vi "Main.vi"() -> ()   [LabVIEW 2013]
doc: "This template is for the Queued Message Handler design pattern.\n\nThe Event Handling Loop generates messages based on user interface actions.\n\nThe Message Handling Loop processes messages generated by the Event Handling Loop, or by other messages. The messages are string values, so new messages can be added easily to the Message Cases case structure in the Message Handling Loop. Each message cluster can also provide an optional value for Message Data, which is a variant that can be converted to whatever message-specific data is required."
uses:
  controls/UI Data.ctl
  support/Message Queue/Enqueue Message (Single).vi
  support/Message Queue/Enqueue Message (Array).vi
  <vilib>/Utility/error.llb/Error Cluster From Error Code.vi
  <vilib>/ErrorRing/Error Ring.xnode
  support/Message Queue/Message Queue.lvlib
  support/User Event - Stop/User Event - Stop.lvlib
panel:
  out "Display <Replace Me>":string
  in  "Do Something Else <Replace Me>":bool
  in  "Do Something <Replace Me>":bool
  in  "Exit":bool
  # "These controls have associated \"Value Changed\" events configured in the Event Structure on the diagram.\n\nReplace them (and reconfigure the Event Structure) with the controls you need for your application."
  # "This template is for the Queued Message Handler design pattern.\n\nSee the block diagram for more information on how to use this template."
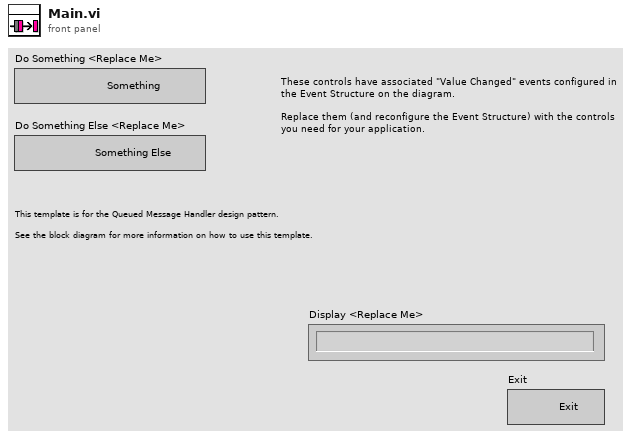
[diagram p1: front panel]
types:
  T1 = typedef "UI Data.ctl" = cluster{"Boolean <Replace Me>":bool, "String <Replace Me>":string, "Numeric <Replace Me>":dbl, "Do Something Ref":refnum<vi>, "Do Something Else Ref":refnum<vi>, "Data Display Ref":refnum<vi>, "Exit Button Ref":refnum<vi>}
  T2 = typedef "Message Queue.lvlib/All Message Queues.ctl" = cluster{"UI":refnum<queue>}
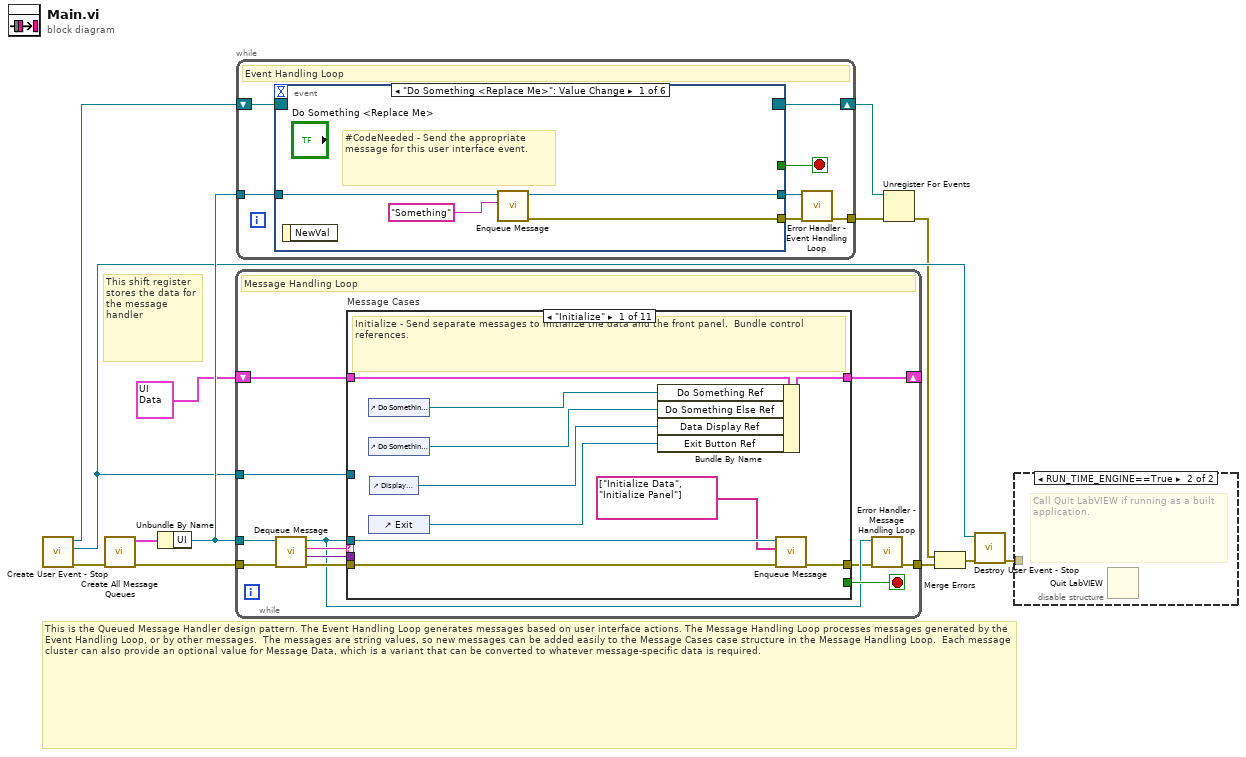
[diagram p0: block diagram]
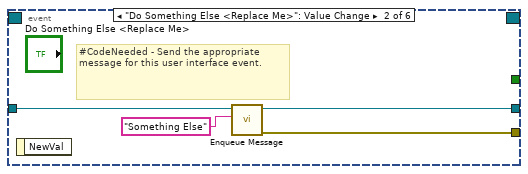
[diagram p3: hidden frame]
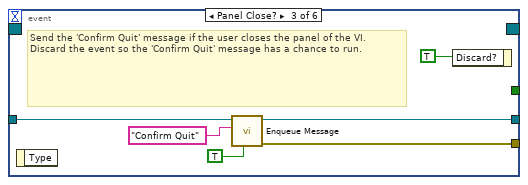
[diagram p4: hidden frame]
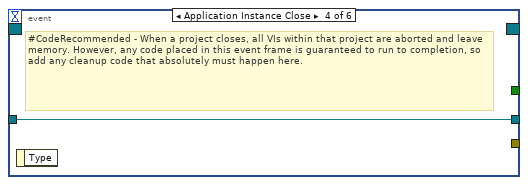
[diagram p5: hidden frame]
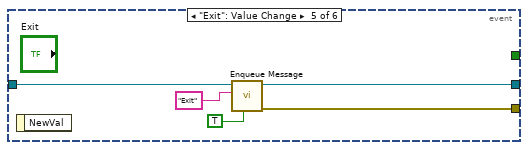
[diagram p6: hidden frame]
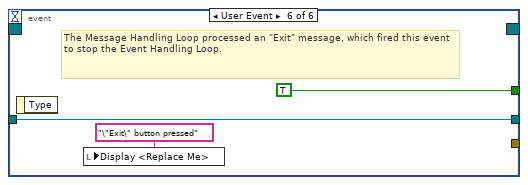
[diagram p7: hidden frame]
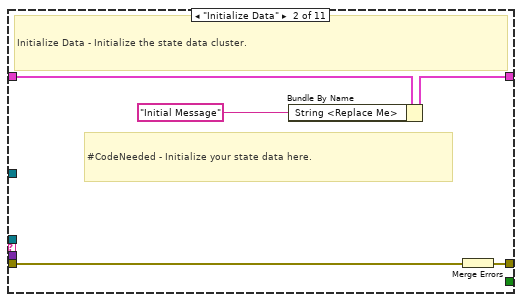
[diagram p8: hidden frame]
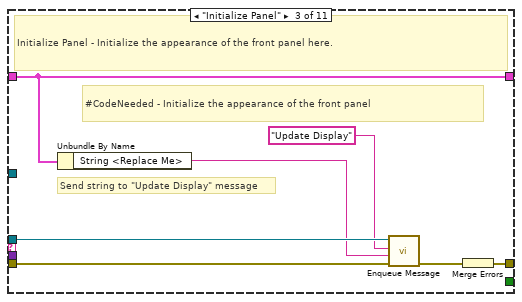
[diagram p9: hidden frame]
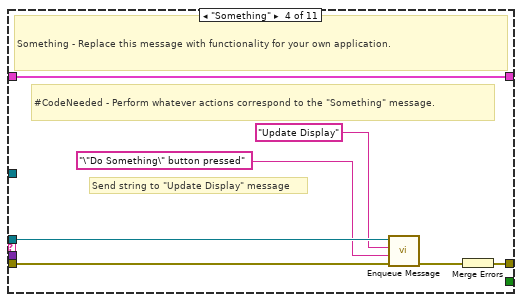
[diagram p10: hidden frame]
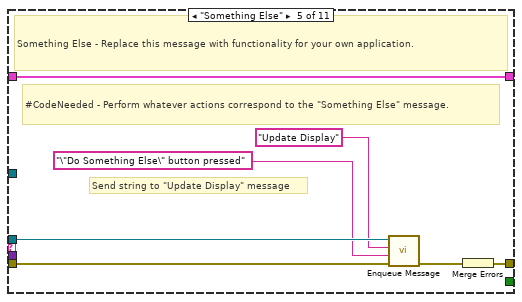
[diagram p11: hidden frame]
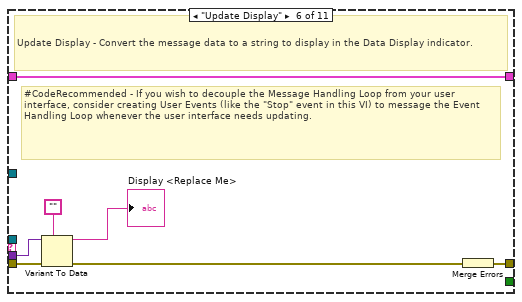
[diagram p12: hidden frame]
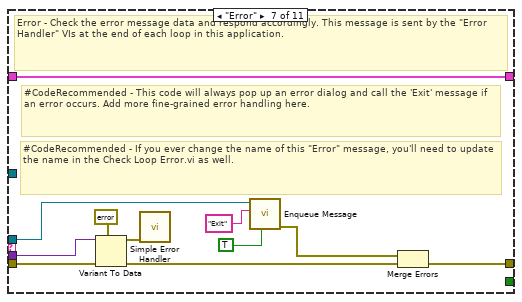
[diagram p13: hidden frame]
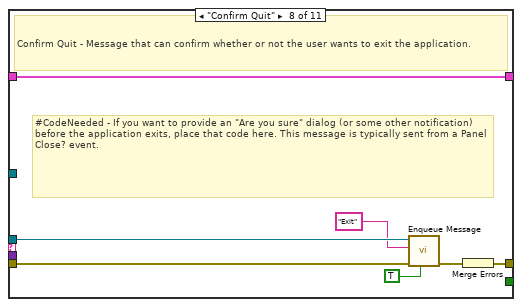
[diagram p14: hidden frame]
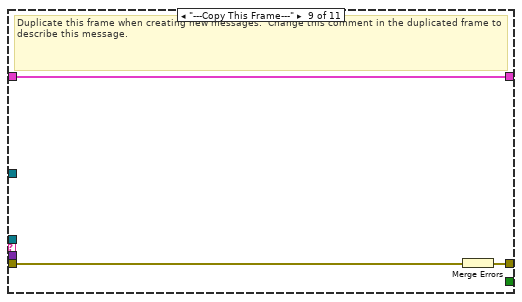
[diagram p15: hidden frame]
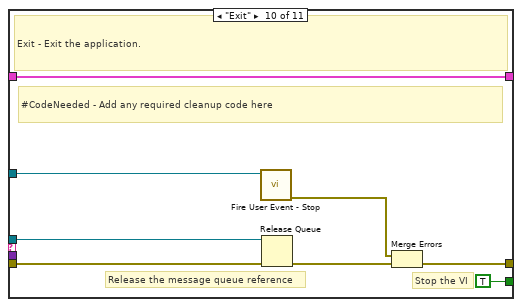
[diagram p16: hidden frame]
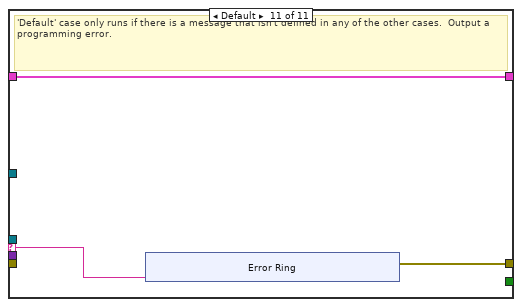
[diagram p17: hidden frame]
diagram:
  # "This is the Queued Message Handler design pattern. The Event Handling Loop generates messages based on user interface actions. The Message Handling Loop processes messages generated by the Event Handling Loop, or by other messages.  The messages are string values, so new messages can be added easily to the Message Cases case structure in the Message Handling Loop.  Each message cluster can also provide an optional value for Message Data, which is a variant that can be converted to whatever message-specific data is required."
  # "This shift register stores the data for the message handler"
  n1 = call "Create User Event - Stop.vi"() -> ("error out"=w8:errorcluster, "User Event - Stop"=w6:refnum<user-event>, "Stop Event Registration Refnum"=w9:refnum<event-registration>)  [unwired: 9 in]
  n2 = call "Create All Message Queues.vi"("error in (no error)"=w8) -> ("error out"=w13:errorcluster, "Message Queues out"=w12:T2)  [unwired: 9 in]
  n3 = Unbundle By Name(w12) -> ("UI"=w10:refnum<queue>)
  n4 = while {
    tunnel: w10 -> [w17]
    shift-right: [w24] -> _
    shift-left: T1 {"Boolean <Replace Me>"=FALSE, "String <Replace Me>"="", "Numeric <Replace Me>"=0.0, "Do Something Ref"=refnum, "Do Something Else Ref"=refnum, "Data Display Ref"=refnum, "Exit Button Ref"=refnum} ("Data Cluster") -> [w25]
    tunnel: w6 -> [w22]
    tunnel: w13 -> [w21]
    tunnel: [w15] -> w11
    stop <- w23 stop-if-true
    # "Message Handling Loop"
    n5 = call "Dequeue Message.vi"("error in (no error)"=w21, "Message Queue"=w17) -> ("error out"=w20:errorcluster, "Message Data"=w18:variant, "Message"=w19:string, "dup Message Queue"=w16:refnum<queue>)  [unwired: 6 in]
    n6 = case "Message Cases" shown="\"Initialize\"" w19 {
      selector: w19 -> [_ _ _ _ _ _ _ _ _ _ w98]
      tunnel: w16 -> [w33 _ w44 w50 w57 _ w71 w82 _ w97 _]
      tunnel: w20 -> [w34 w40 w45 w52 w59 w66 w79 w86 w89 w92 _]
      tunnel: [w35 w36 w46 w53 w60 w67 w72 w84 w87 w93 w99] -> w14
      tunnel: w25 -> [w32 w39 w47 w54 w61 w68 w78 w85 w88 w96 w100]
      tunnel: [w31 w38 w47 w54 w61 w68 w78 w85 w88 w96 w100] -> w24
      tunnel: [_ _ _ _ _ _ _ _ _ TRUE _] -> w23
      tunnel: w18 -> [_ _ _ _ _ w65 w77 _ _ _ _]
      tunnel: w22 -> [_ _ _ _ _ _ _ _ _ w91 _]
      frame "Initialize" {
        # "Initialize - Send separate messages to initialize the data and the front panel.  Bundle control references."
        n7 = control-ref of="Do Something <Replace Me>"() -> (w30:refnum<vi>)
        n8 = control-ref of="Do Something Else <Replace Me>"() -> (w29:refnum<vi>)
        n9 = control-ref of="Exit"() -> (w27:refnum<vi>)
        n10 = control-ref of="Display <Replace Me>"() -> (w28:refnum<vi>)
        n11 = Bundle By Name(cluster=w32, "Do Something Ref"=w30, "Do Something Else Ref"=w29, "Data Display Ref"=w28, "Exit Button Ref"=w27) -> (w31:T1)
        n12 = call-poly "Enqueue Message.vi"("error in (no error)"=w34, "Message Array"=string[] ["Initialize Data", "Initialize Panel"], "Message Queue"=w33) -> ("error out"=w35:errorcluster)  [unwired: 7 in, 1 out]
      }
      frame "Initialize Data" {
        # "#CodeNeeded - Initialize your state data here."
        # "Initialize Data - Initialize the state data cluster."
        n13 = Bundle By Name(cluster=w39, "String <Replace Me>"="Initial Message" ("Initial Message")) -> (w38:T1)
        n14 = Merge Errors(w40) -> (w36:errorcluster)
      }
      frame "Initialize Panel" {
        # "Send string to \"Update Display\" message"
        # "#CodeNeeded - Initialize the appearance of the front panel"
        # "Initialize Panel - Initialize the appearance of the front panel here."
        n15 = Unbundle By Name(w47) -> ("String <Replace Me>"=w41:string)
        n16 = call-poly "Enqueue Message.vi"("error in (no error)"=w45, "Message Data"=w41, "Message"="Update Display", "Message Queue"=w44) -> ("error out"=w43:errorcluster)  [unwired: 6 in, 1 out]
        n17 = Merge Errors(w43) -> (w46:errorcluster)
      }
      frame "Something" {
        # "Send string to \"Update Display\" message"
        # "#CodeNeeded - Perform whatever actions correspond to the \"Something\" message."
        # "Something - Replace this message with functionality for your own application."
        n18 = call-poly "Enqueue Message.vi"("error in (no error)"=w52, "Message Data"="\"Do Something\" button pressed" ("\"Do Something\" button pressed"), "Message"="Update Display", "Message Queue"=w50) -> ("error out"=w51:errorcluster)  [unwired: 6 in, 1 out]
        n19 = Merge Errors(w51) -> (w53:errorcluster)
      }
      frame "Something Else" {
        # "Send string to \"Update Display\" message"
        # "#CodeNeeded - Perform whatever actions correspond to the \"Something Else\" message."
        # "Something Else - Replace this message with functionality for your own application."
        n20 = call-poly "Enqueue Message.vi"("error in (no error)"=w59, "Message Data"="\"Do Something Else\" button pressed" ("\"Do Something Else\" button pressed"), "Message"="Update Display", "Message Queue"=w57) -> ("error out"=w58:errorcluster)  [unwired: 6 in, 1 out]
        n21 = Merge Errors(w58) -> (w60:errorcluster)
      }
      frame "Update Display" {
        # "#CodeRecommended - If you wish to decouple the Message Handling Loop from your user interface, consider creating User Events (like the \"Stop\" event in this VI) to message the Event Handling Loop whenever the user interface needs updating."
        # "Update Display - Convert the message data to a string to display in the Data Display indicator."
        n22 = Variant To Data(error in=w66, type="", Variant=w65) -> (data=→"Display <Replace Me>":string, error out=w63:errorcluster)
        n23 = Merge Errors(w63) -> (w67:errorcluster)
      }
      frame "Error" {
        # "#CodeRecommended - If you ever change the name of this \"Error\" message, you'll need to update the name in the Check Loop Error.vi as well."
        # "#CodeRecommended - This code will always pop up an error dialog and call the 'Exit' message if an error occurs. Add more fine-grained error handling here."
        # "Error - Check the error message data and respond accordingly. This message is sent by the \"Error Handler\" VIs at the end of each loop in this application."
        n24 = Variant To Data(error in=w79, type=errorcluster {"status"=FALSE, "code"=0, "source"=""} ("error constant"), Variant=w77) -> (data=w75:errorcluster, error out=w74:errorcluster)
        n25 = call <vilib>:"Simple Error Handler.vi"("error in (no error)"=w75) -> ()  [unwired: 4 in, 5 out]
        n26 = call-poly "Enqueue Message.vi"("Priority Message? (F)"=TRUE, "Message"="Exit", "Message Queue"=w71) -> ("error out"=w73:errorcluster)  [unwired: 7 in, 1 out]
        n27 = Merge Errors(w73, w74) -> (w72:errorcluster)
      }
      frame "Confirm Quit" {
        # "#CodeNeeded - If you want to provide an \"Are you sure\" dialog (or some other notification) before the application exits, place that code here. This message is typically sent from a Panel Close? event."
        # "Confirm Quit - Message that can confirm whether or not the user wants to exit the application."
        n28 = call-poly "Enqueue Message.vi"("Priority Message? (F)"=TRUE, "error in (no error)"=w86, "Message"="Exit", "Message Queue"=w82) -> ("error out"=w83:errorcluster)  [unwired: 6 in, 1 out]
        n29 = Merge Errors(w83) -> (w84:errorcluster)
      }
      frame "---Copy This Frame---" {
        # "Duplicate this frame when creating new messages.  Change this comment in the duplicated frame to describe this message."
        n30 = Merge Errors(w89) -> (w87:errorcluster)
      }
      frame "Exit" {
        # "Stop the VI"
        # "Release the message queue reference"
        # "#CodeNeeded - Add any required cleanup code here"
        # "Exit - Exit the application."
        n31 = call "Fire User Event - Stop.vi"("User Event - Stop"=w91) -> ("error out"=w90:errorcluster)  [unwired: 10 in]
        n32 = Release Queue(queue=w97, error in (no error)=w92) -> (error out=w94:errorcluster)  [unwired: 1 in, 2 out]
        n33 = Merge Errors(w90, w94) -> (w93:errorcluster)
      }
      frame Default {
        # "'Default' case only runs if there is a message that isn't defined in any of the other cases.  Output a programming error."
        n34 = xnode "Error Ring"("parameter 0"=w98) -> ("error out"=w99:errorcluster)
      }
    }
    n35 = call "Error Handler - Message Handling Loop.vi"("error in (no error)"=w14, "Message Queue"=w16) -> ("dup error in"=w15:errorcluster)  [unwired: 8 in, 1 out]
  }
  n36 = while {
    tunnel: w10 -> [w114]
    shift-right: [w112] -> w4
    shift-left: w9 -> [w113]
    tunnel: [w108] -> w1
    stop <- w110 stop-if-true
    # "Event Handling Loop"
    n37 = event shown="[0] \"Do Something <Replace Me>\": Value Change" {
      selector: w113 -> [_ _ _ _ _ _]
      dyn-events: [_ _ _ _ _ _] -> w112
      timeout: _ -> [_ _ _ _ _ _]
      tunnel: [_ _ _ _ _ TRUE ("Discard?")] -> w110
      tunnel: w114 -> [w118 w122 w127 w129 w134 w137]
      tunnel: [w115 w119 w126 _ w133 _] -> w111
      tunnel: [w117 w121 w125 w129 w132 w137] -> w109
      event "Do Something <Replace Me>": Value Change {
        # "#CodeNeeded - Send the appropriate message for this user interface event."
        n38 = event-data() -> ()  [unwired: 1 in, 1 out]
        n39 = call-poly "Enqueue Message.vi"("Message"="Something", "Message Queue"=w118) -> ("error out"=w115:errorcluster, "dup Message Queue"=w117:refnum<queue>)  [unwired: 8 in]
      }
      event "Do Something Else <Replace Me>": Value Change {
        # "#CodeNeeded - Send the appropriate message for this user interface event."
        n40 = event-data() -> ()  [unwired: 1 in, 1 out]
        n41 = call-poly "Enqueue Message.vi"("Message"="Something Else", "Message Queue"=w122) -> ("error out"=w119:errorcluster, "dup Message Queue"=w121:refnum<queue>)  [unwired: 8 in]
      }
      event Panel Close? {
        # "Send the 'Confirm Quit' message if the user closes the panel of the VI. Discard the event so the 'Confirm Quit' message has a chance to run."
        n42 = event-data() -> ()  [unwired: 1 in, 1 out]
        n43 = call-poly "Enqueue Message.vi"("Priority Message? (F)"=TRUE, "Message"="Confirm Quit", "Message Queue"=w127) -> ("error out"=w126:errorcluster, "dup Message Queue"=w125:refnum<queue>)  [unwired: 7 in]
        n44 = event-data("Discard?"=TRUE) -> ()  [unwired: 1 in, 1 out]
      }
      event Application Instance Close {
        # "#CodeRecommended - When a project closes, all VIs within that project are aborted and leave memory. However, any code placed in this event frame is guaranteed to run to completion, so add any cleanup code that absolutely must happen here."
        n45 = event-data() -> ()  [unwired: 1 in, 1 out]
      }
      event "Exit": Value Change {
        n46 = event-data() -> ()  [unwired: 1 in, 1 out]
        n47 = call-poly "Enqueue Message.vi"("Priority Message? (F)"=TRUE, "Message"="Exit", "Message Queue"=w134) -> ("error out"=w133:errorcluster, "dup Message Queue"=w132:refnum<queue>)  [unwired: 7 in]
      }
      event User Event {
        # "The Message Handling Loop processed an \"Exit\" message, which fired this event to stop the Event Handling Loop."
        n48 = event-data() -> ()  [unwired: 1 in, 1 out]
        n49 = local write "Display <Replace Me>"("\"Exit\" button pressed" ("VI Stopped")) -> ()
      }
    }
    n50 = call "Error Handler - Event Handling Loop.vi"("error in (no error)"=w111, "Message Queue"=w109) -> ("dup error in"=w108:errorcluster)  [unwired: 8 in, 1 out]
  }
  n51 = Unregister For Events(event registration refnum=w4, error in=w1) -> (error out=w5:errorcluster)
  n52 = Merge Errors(w5, w11) -> (w7:errorcluster)
  n53 = call "Destroy User Event - Stop.vi"("error in (no error)"=w7, "User Event - Stop"=w6) -> ("error out"=w2:errorcluster)  [unwired: 9 in]
  n54 = disable-structure shown="RUN_TIME_ENGINE==True" {
    disable-tunnel: w2 -> [_ _]
    frame condition #0 (active) {
    }
    frame condition #1 {
      # "Call Quit LabVIEW if running as a built application."
      n55 = Quit LabVIEW() -> ()  [unwired: 1 in]
    }
  }
